vi "Protocol_Parsor.vi"() -> ()   [LabVIEW 2018]
panel:
  out "연결된 문자열":string
  out "길이":i32[](array[numeric])
  out "기계이름 다음 값을 가지고 옮":string
  out "통신으로 받은 데이터 크기":i32
  out "배열":string[](array[string])
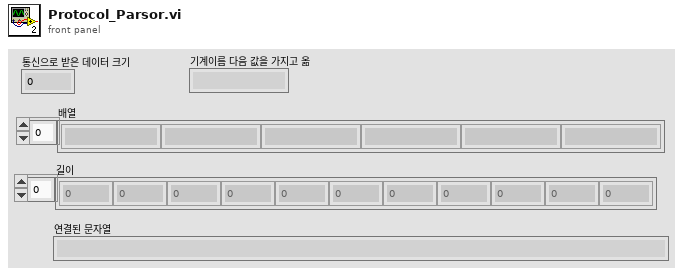
[diagram p1: front panel]
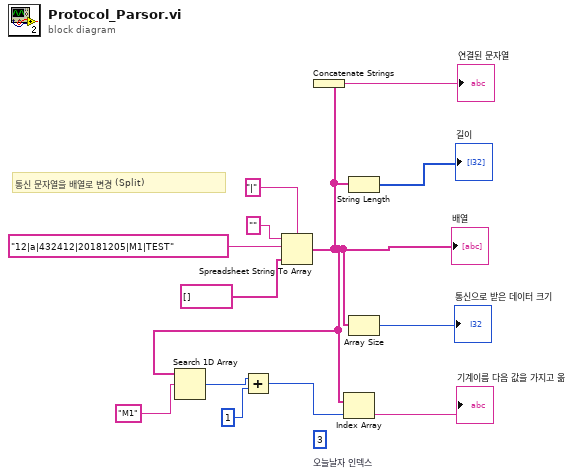
[diagram p0: block diagram]
diagram:
  (unwired) 3  # 오늘날자 인덱스
  # "통신 문자열을 배열로 변경 (Split)"
  n1 = Spreadsheet String To Array ("스프레드시트 문자열을 배열로")(delimiter (Tab)="|", format string="" ("포맷 문자열"), spreadsheet string="12|a|432412|20181205|M1|TEST", array type (2D Dbl)=string[] []) -> (array=w2:string[])
  "배열" <- w2
  n2 = Search 1D Array(1D array=w2, element="M1") -> (index of element=w5:i32)  [unwired: 1 in]
  n3 = Add(x=w5, y=1) -> (x+y=w4:i32)
  n4 = Concatenate Strings(w2) -> (→"연결된 문자열":string)
  n5 = Index Array(array=w2, index=w4) -> (element=→"기계이름 다음 값을 가지고 옮":string)
  n6 = String Length(string=w2) -> (length=→"길이":i32[])
  n7 = Array Size(array=w2) -> (size(s)=→"통신으로 받은 데이터 크기":i32)
